vi "gas flow controller -- Pgg3.vi"(5 "gas flow, %":dbl=11.0, 6 "action":T3=enum."stop UP/DOWN", 7 "heater":dbl=11.0, 8 "gas flow controller ref in":refnum<vi>, 10 "seconds":dbl=1.0) -> (0 "gas flow controller out":T1={"UP step (%)"=10.0, "ramp DOWN"=TRUE, "ramp UP"=TRUE, "idle"=TRUE, "UP time (min)"=10.0, "ramp step (%)"=10.0, "check (min)"=10.0, "DOWN step (%)"=10.0, "DOWN time (min)"=10.0, "to"=10.0, "last (min)"=10.0, "below"=TRUE, "above"=TRUE, "Control Gas"=TRUE, "upper"=10.0, "lower"=10.0, "heater"=10.0, "in range"=TRUE, "gas, %"=10.0, "ramp Up progress"={"(total # of ramp steps)"=30, "ramp time step (sec)"=120, "steps so far"=0, "state"=enum."ramp down"}, "ramp Down progress"={"(total # of ramp steps)"=30, "ramp time step (sec)"=120, "steps so far"=0, "state"=enum."ramp down"}, "state"=enum."normal", "set gas"=TRUE})   [LabVIEW 2015]
uses:
  gas flow controller action.ctl
  gas flow controller control -- Pgg2.ctl
  gas flow control - progress.ctl
  gas flow controller state.ctl
  stack action -- control.ctl
  itc 503 box - control.ctl
  Q - not nan -- real.vi
  Q - not nan -- integer.vi
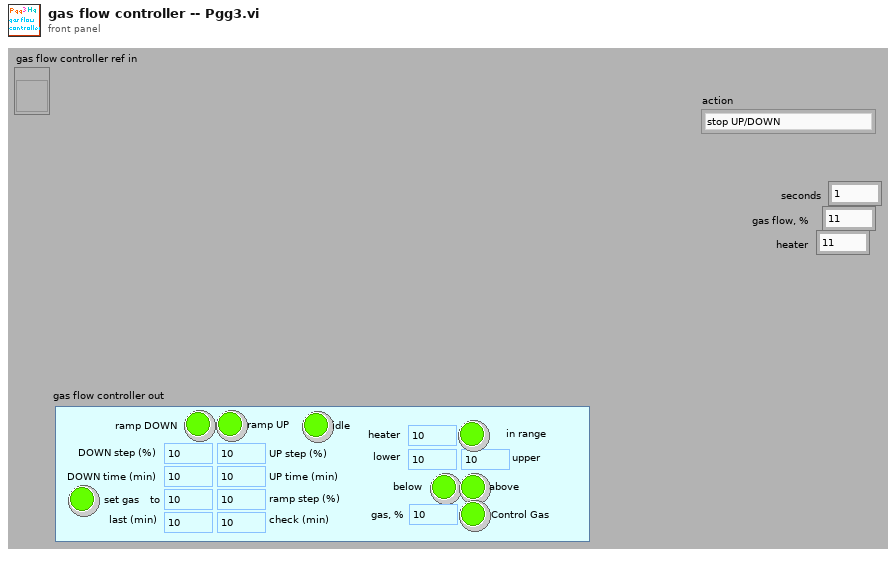
[diagram p1: front panel]
types:
  T1 = typedef "gas flow controller control -- Pgg2.ctl" = cluster{"UP step (%)":dbl, "ramp DOWN":bool, "ramp UP":bool, "idle":bool, "UP time (min)":dbl, "ramp step (%)":dbl, "check (min)":dbl, "DOWN step (%)":dbl, "DOWN time (min)":dbl, "to":dbl, "last (min)":dbl, "below":bool, "above":bool, "Control Gas":bool, "upper":dbl, "lower":dbl, "heater":dbl, "in range":bool, "gas, %":dbl, "ramp Up progress":T2, "ramp Down progress":T2, "state":enum16{"normal", "ramp up", "ramp down"}, "set gas":bool}
  T2 = typedef "gas flow control - progress.ctl" = cluster{"(total # of ramp steps)":i32, "ramp time step (sec)":i32, "steps so far":i32, "state":enum16{"normal", "ramp up", "ramp down"}}
  T3 = typedef "gas flow controller action.ctl" = enum16{"check", "force UP", "stop UP/DOWN", "force DOWN", "init", "set gas to", "turn off", "turn on", "idle", "update parameters", "parse", "set gas"}
  T4 = typedef "gas flow controller state.ctl" = enum16{"normal", "ramp up", "ramp down"}
  T5 = typedef "stack action -- control.ctl" = enum16{"push", "pop", "check", "init"}
  T6 = typedef "itc 503 box - control.ctl" = enum16{"heater manual and zero", "heater auto", "upload D", "upload I", "upload P", "shut off", "init", "read sweep table", "disable", "enable", "read state", "set gas to", "stop sweep", "start sweep", "test", "set temperature to", "write sweep table", "-void", "set heater to"}
  T7 = typedef "comparison control.ctl" = enum16{"not a number", "above", "in range", "below"}
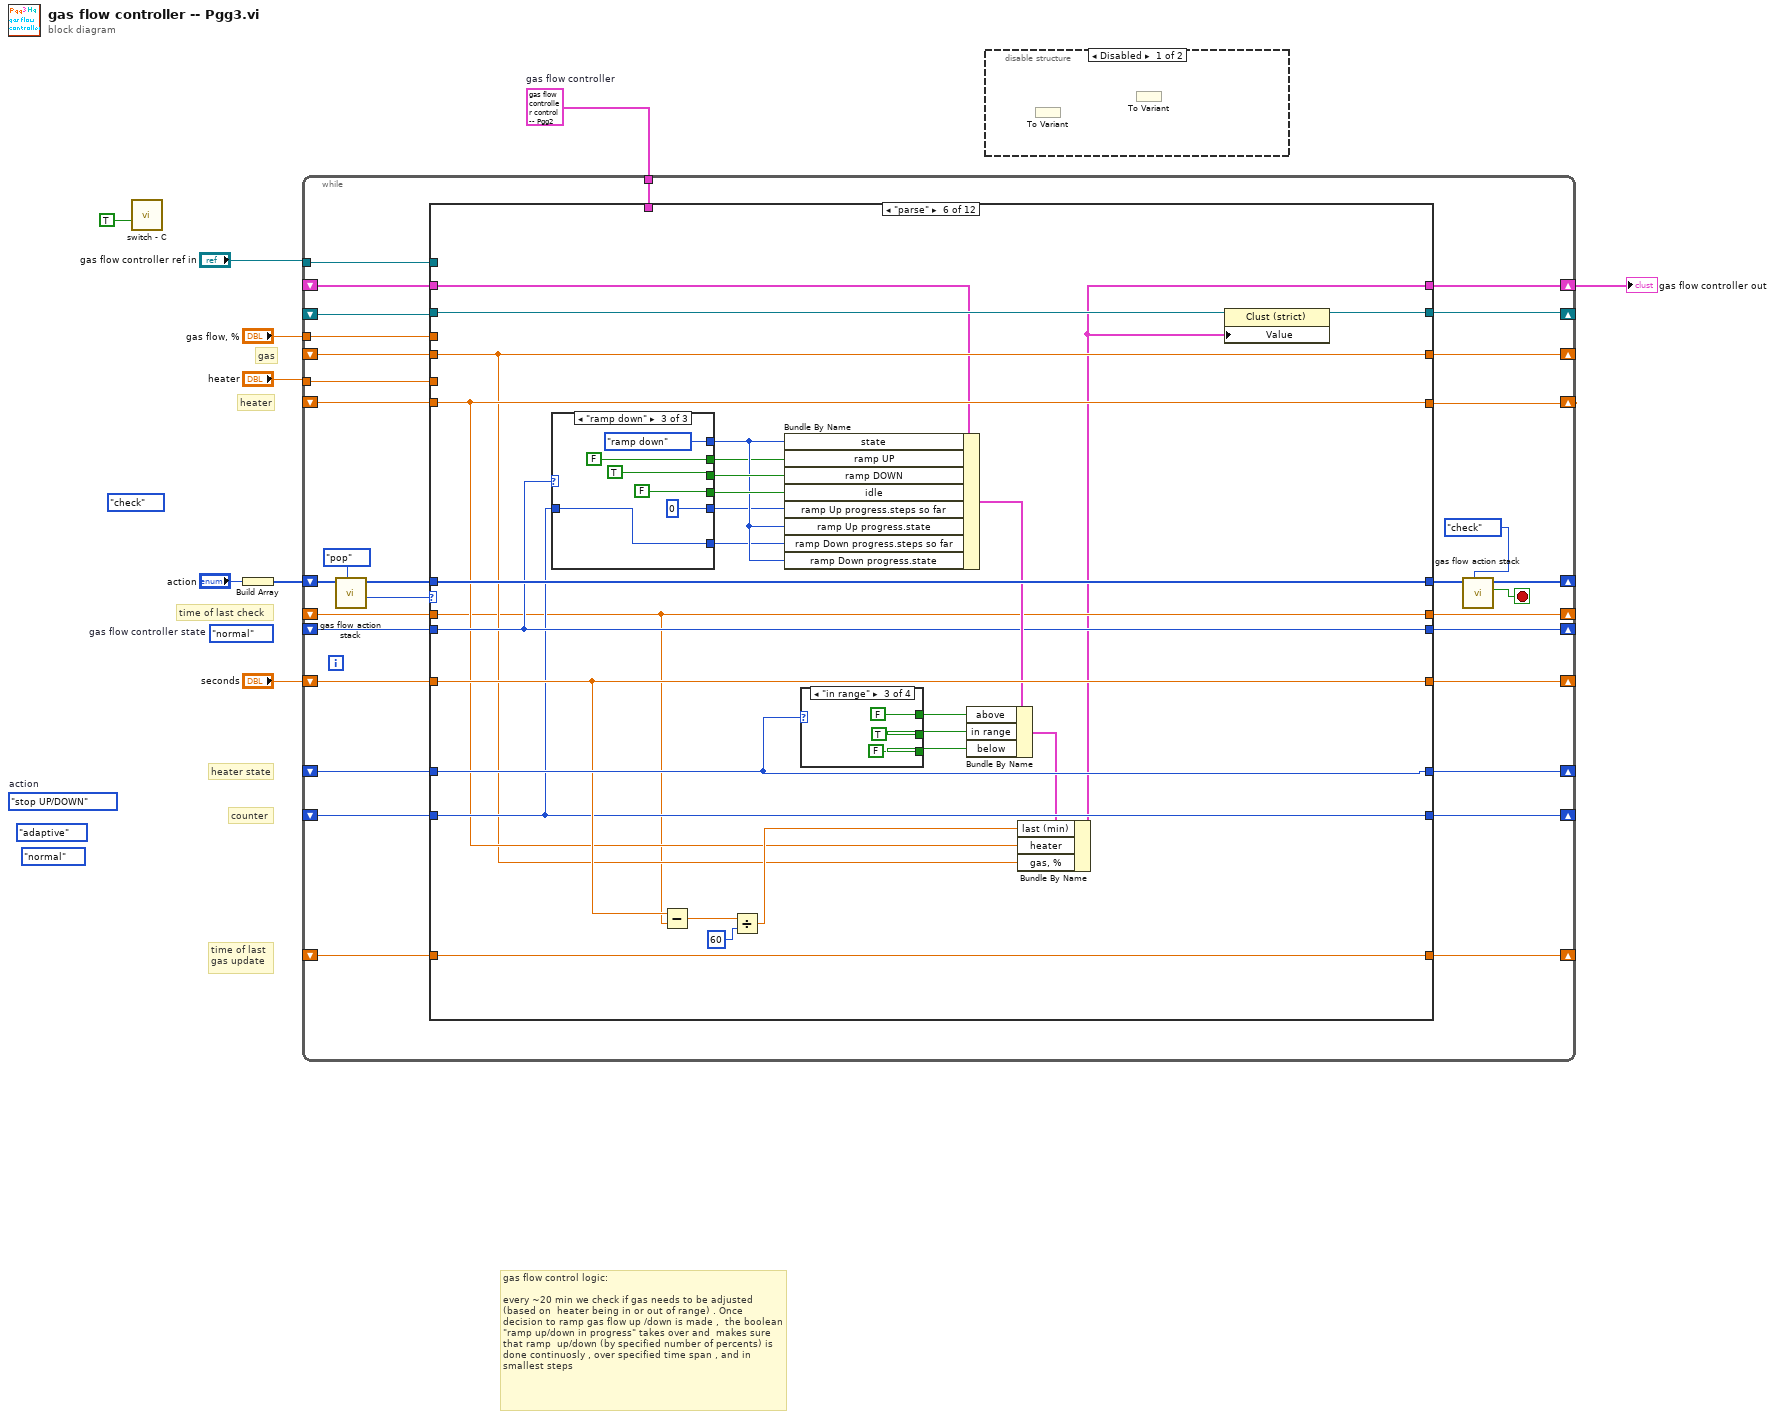
[diagram p0: block diagram]
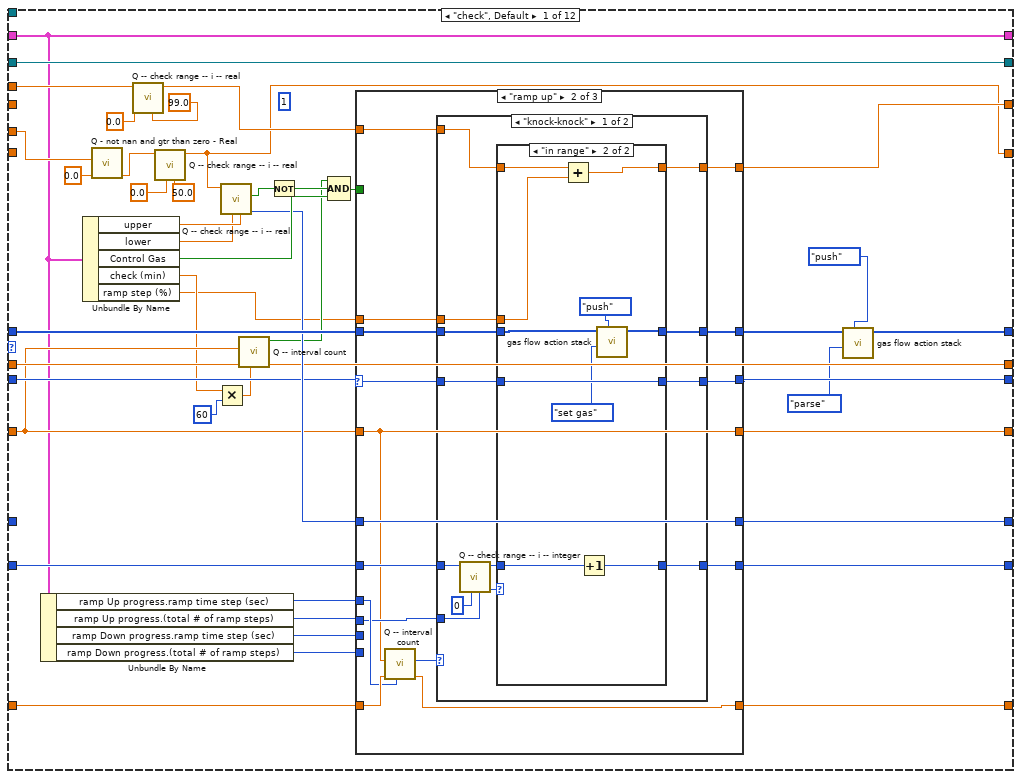
[diagram p3: hidden frame]
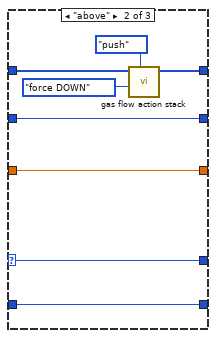
[diagram p6: hidden frame]
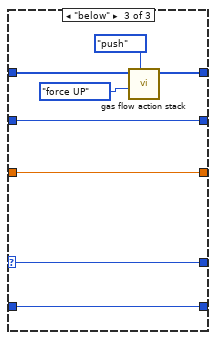
[diagram p7: hidden frame]
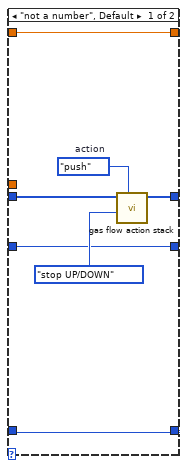
[diagram p8: hidden frame]
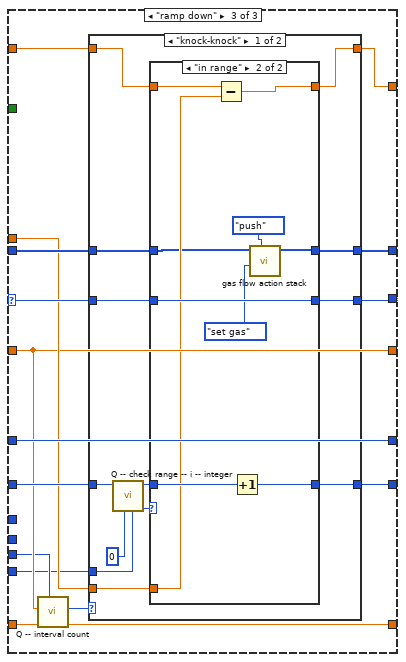
[diagram p10: hidden frame]
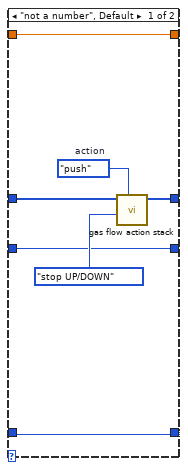
[diagram p11: hidden frame]
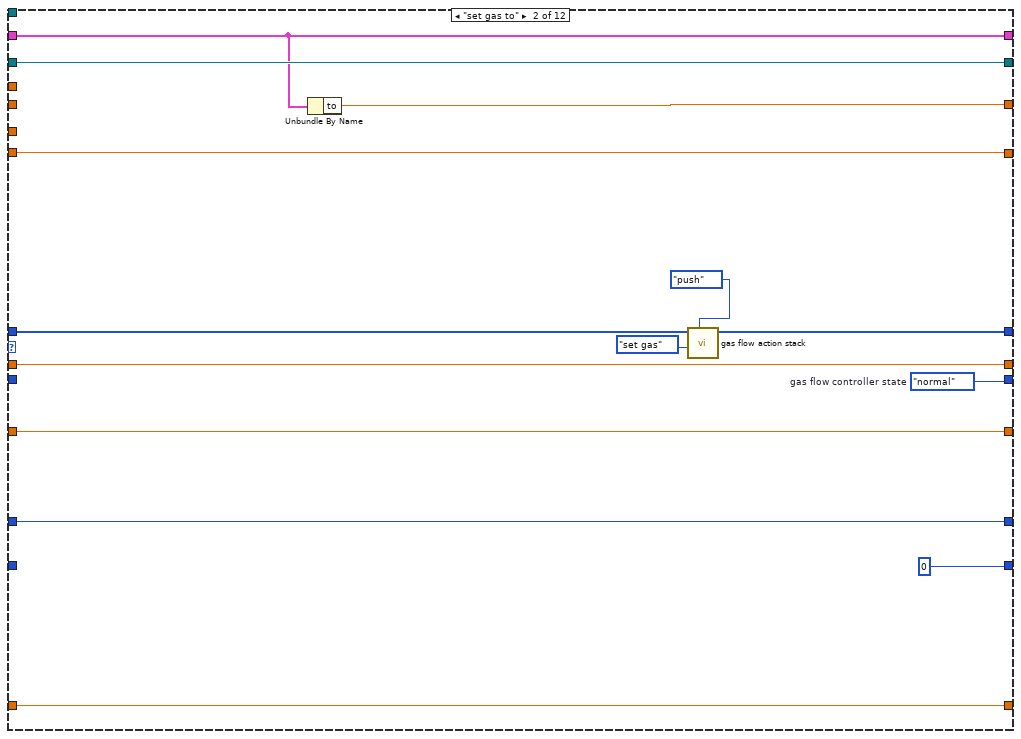
[diagram p13: hidden frame]
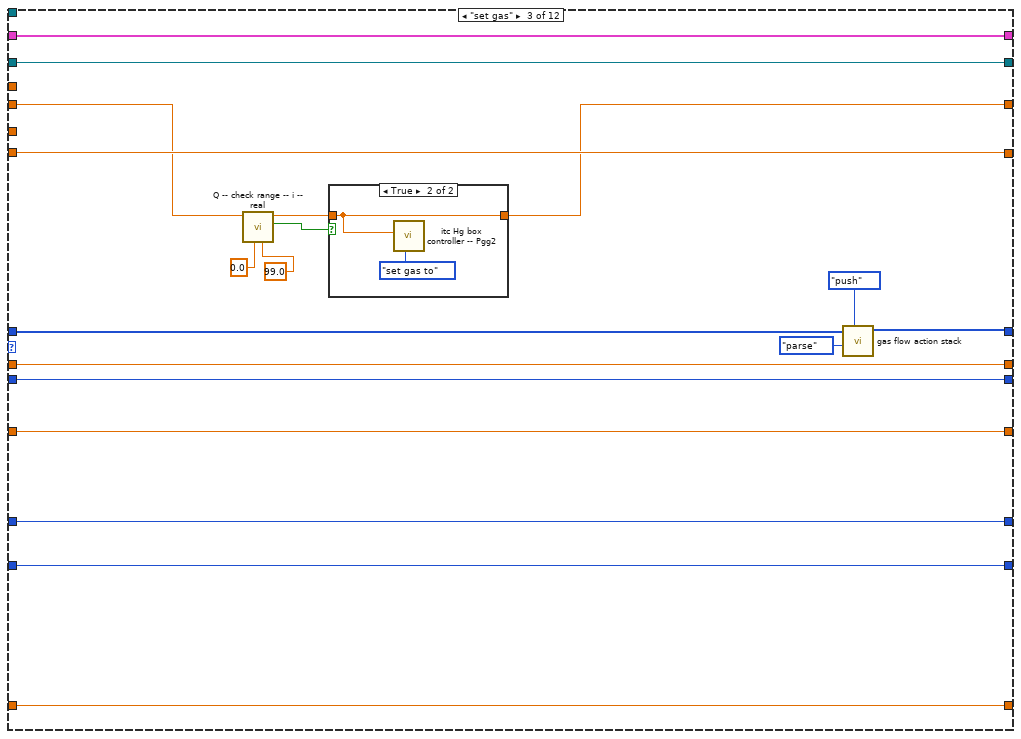
[diagram p14: hidden frame]
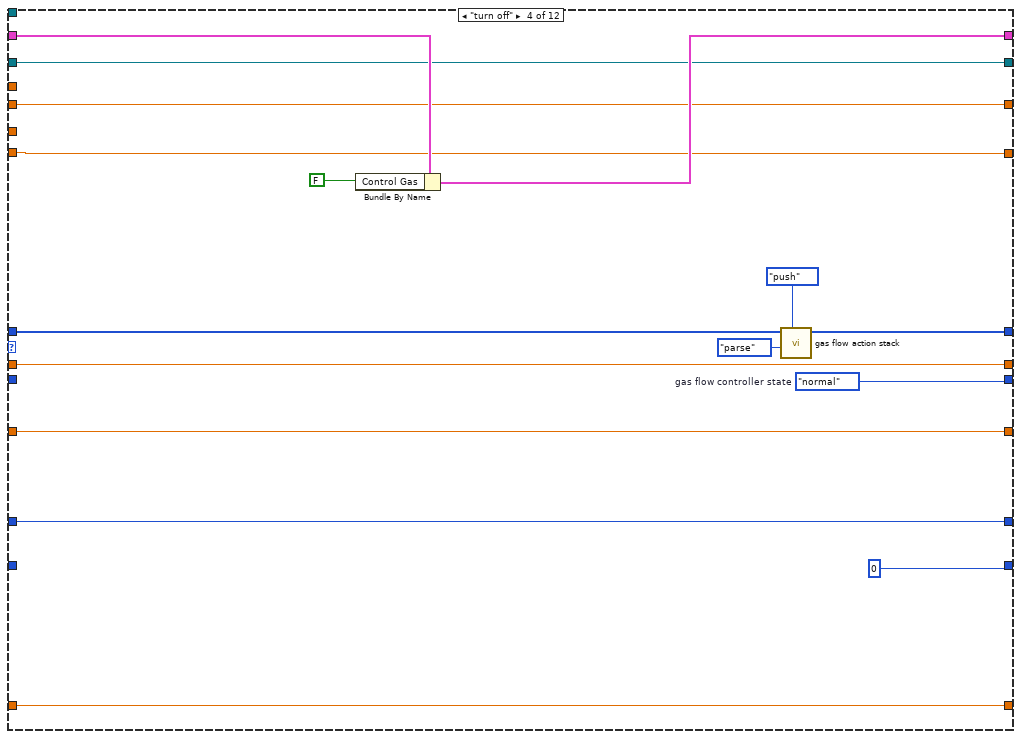
[diagram p16: hidden frame]
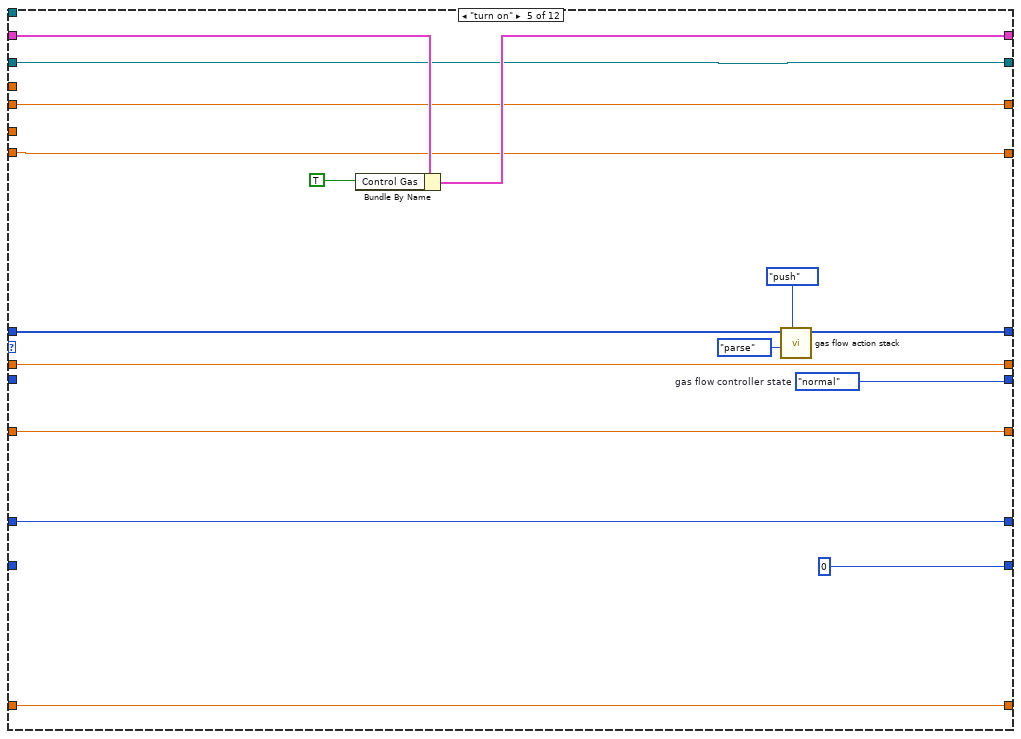
[diagram p17: hidden frame]
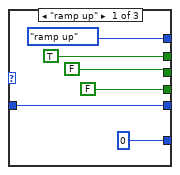
[diagram p18: hidden frame]
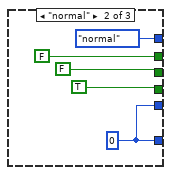
[diagram p19: hidden frame]
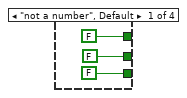
[diagram p20: hidden frame]
diagram:
  (unwired) gas_flow_controller_action."check" ("action")
  w2 = T1 {"UP step (%)"=0.5, "ramp DOWN"=FALSE, "ramp UP"=FALSE, "idle"=FALSE, "UP time (min)"=20.0, "ramp step (%)"=0.1, "check (min)"=3.0, "DOWN step (%)"=0.5, "DOWN time (min)"=20.0, "to"=1.0, "last (min)"=0.0, "below"=FALSE, "above"=FALSE, "Control Gas"=FALSE, "upper"=7.0, "lower"=3.0, "heater"=0.0, "in range"=TRUE, "gas, %"=1.0, "ramp Up progress"={"(total # of ramp steps)"=30, "ramp time step (sec)"=120, "steps so far"=0, "state"=enum."ramp down"}, "ramp Down progress"={"(total # of ramp steps)"=30, "ramp time step (sec)"=120, "steps so far"=0, "state"=enum."ramp down"}, "state"=enum."ramp down", "set gas"=FALSE}  # gas flow controller
  (unwired) enum16{"normal", "ramp up", "ramp down"}."normal" ("state")
  (unwired) enum16{"first time", "uniform", "adaptive"}."adaptive" ("mode")
  (unwired) gas_flow_controller_state."normal"  # gas flow controller state
  (unwired) gas_flow_controller_action."stop UP/DOWN"  # action
  # "heater"
  # "time of last\ngas update"
  # "counter"
  # "heater state"
  # "gas"
  # "gas flow control logic: \n\nevery ~20 min we check if gas needs to be adjusted  (based on  heater being in or out of range) . Once  decision to ramp gas flow up /down is made ,  the boolean \"ramp up/down in progress\" takes over and  makes sure that ramp  up/down (by specified number of percents) is done continuosly , over specified time span , and in smallest steps"
  # "time of last check"
  n1 = call "switch - C.vi"("switch"=TRUE) -> ()  [unwired: 10 in, 1 out]
  n2 = Build Array("action") -> (w5:T3[])
  n3 = while {
    shift-right: [w11] -> w3
    shift-left: _ -> [w41]
    shift-right: [w23] -> _
    shift-left: _ -> [w20]
    tunnel: "gas flow, %" -> [w24]
    tunnel: "heater" -> [w40]
    shift-right: [w38] -> _
    shift-left: _ -> [w37]
    shift-right: [w36] -> _
    shift-left: _ -> [w35]
    shift-right: [w29] -> _
    shift-left: w5 -> [w34]
    shift-right: [w25] -> _
    shift-left: _ -> [w26]
    shift-right: [w22] -> _
    shift-left: _ -> [w21]
    shift-right: [w18] -> _
    shift-left: "seconds" -> [w39]
    shift-right: [w19] -> _
    shift-left: _ -> [w13]
    shift-right: [w17] -> _
    shift-left: _ -> [w16]
    shift-right: [w15] -> _
    shift-left: _ -> [w14]
    tunnel: "gas flow controller ref in" -> [w12]
    tunnel: w2 -> [w10]
    stop <- w27 stop-if-true
    n4 = call "gas flow action stack.vi"("action"=stack_action_--_control."pop", "command stack"=w34) -> ("selector out"=w33:T3, "command stack out"=w31:T3[])  [unwired: 7 in, 1 out]
    n5 = case shown="\"parse\"" w33 {
      tunnel: [w44 w238 w250 w283 w299 w304 w360 w411 w417 w437 w454 w469] -> w11
      tunnel: w41 -> [w44 w238 w250 w286 w302 w305 w369 w411 _ w437 w454 w469]
      tunnel: w40 -> [w49 _ _ _ _ _ _ _ _ _ _ _]
      tunnel: w39 -> [w66 w241 w265 w276 w292 w326 w375 w408 w421 w438 w443 w461]
      tunnel: [w55 w249 w268 w272 w288 w329 w380 w412 w420 w436 w455 w470] -> w38
      tunnel: w37 -> [w55 w249 w268 w272 w288 w308 w368 w412 _ w436 w455 w470]
      tunnel: [w75 w248 w267 w285 w301 w306 w378 w415 w431 w442 w445 w459] -> w36
      tunnel: w35 -> [w77 w248 w267 w285 w301 w306 w378 w415 w431 w442 _ _]
      tunnel: [w59 w245 w260 w281 w297 w330 w377 w403 w424 w435 w448 w463] -> w30
      tunnel: w31 -> [w80 w237 w259 w280 w296 w330 w377 w404 w425 w435 w449 w464]
      tunnel: w26 -> [w78 _ w257 _ _ w317 w376 _ _ w432 _ _]
      tunnel: [w72 w247 w257 w284 w300 w317 w376 w414 w430 w432 w457 w472] -> w25
      tunnel: w24 -> [w71 _ _ _ _ _ _ _ _ _ _ _]
      tunnel: [w51 w246 w251 w278 w294 w309 w370 w410 w428 w441 w453 w468] -> w23
      tunnel: [w50 w242 w266 w277 w293 w310 w371 w409 w427 w440 w452 w467] -> w22
      tunnel: w21 -> [_ w242 w266 w277 w293 w310 w371 w409 w427 w440 w452 w467]
      tunnel: w20 -> [_ _ w253 w278 w294 w309 w370 w410 w428 w441 w453 w468]
      tunnel: [w56 w240 w264 w275 w291 w328 w374 w407 w422 w439 w451 w466] -> w19
      tunnel: [w57 w241 w265 w276 w292 w326 w375 w408 w421 w438 w443 w461] -> w18
      tunnel: [w65 w239 w262 w274 w290 w327 w372 w405 w421 w434 w445 w459] -> w17
      tunnel: w16 -> [w64 w239 w262 w274 w290 w327 w372 w405 _ w434 w444 w458]
      tunnel: [w63 0 w263 0 0 w314 w373 0 0 w433 0 0] -> w15
      tunnel: w14 -> [w62 _ w263 _ _ w314 w373 _ _ w433 _ _]
      tunnel: w13 -> [_ w240 w264 w275 w291 w328 w374 w407 w422 w439 w451 w466]
      tunnel: w12 -> [_ _ _ _ _ _ _ _ w419 _ _ _]
      tunnel: w10 -> [_ _ _ _ _ _ w361 _ w416 _ _ _]
      frame "check", Default {
        (unwired) 1
        n6 = Unbundle By Name(w44) -> ("ramp Up progress.ramp time step (sec)"=w54:i32, "ramp Up progress.(total # of ramp steps)"=w53:i32, "ramp Down progress.ramp time step (sec)"=w46:i32, "ramp Down progress.(total # of ramp steps)"=w45:i32)
        n7 = Unbundle By Name(w44) -> ("upper"=w84:dbl, "lower"=w83:dbl, "Control Gas"=w86:bool, "check (min)"=w43:dbl, "ramp step (%)"=w42:dbl)
        n8 = call "Q - not nan and gtr than zero - Real.vi"("default"=0.0 ("y"), "Numeric"=w49) -> ("out"=w47:dbl)  [unwired: 8 in, 1 out]
        n9 = call "Q -- check range -- i -- real.vi"("upper"=99.0 ("y"), "lower"=0.0 ("y"), "number"=w71) -> ("number in range"=w52:dbl)  [unwired: 6 in, 2 out]
        n10 = call "Q -- check range -- i -- real.vi"("upper"=50.0 ("y"), "lower"=0.0 ("y"), "number"=w47) -> ("number in range"=w50:dbl)  [unwired: 6 in, 2 out]
        n11 = Multiply(x=w43, y=60) -> (x*y=w76:dbl)
        n12 = call "Q -- check range -- i -- real.vi"("upper"=w84, "lower"=w83, "number"=w50) -> ("selector"=w79:T7, "in range?"=w82:bool)  [unwired: 6 in, 1 out]
        n13 = call "Q -- interval count.vi"("interval (sec)"=w76, "last time (sec)"=w77, "current time (sec)"=w66) -> ("last time out (sec)"=w75:dbl, "tic"=w73:bool)  [unwired: 5 in, 2 out]
        n14 = Not(x=w82) -> (.not. x?=w85:bool)
        n15 = Compound Arithmetic op=AND(w73, w85, w86) -> (w81:bool)
        n16 = case shown="\"ramp up\"" w78 {
          selector: w78 -> [w92 w144 w194]
          tunnel: w81 -> [w99 _ _]
          tunnel: w66 -> [w98 w136 w188]
          tunnel: [w87 w150 w200] -> w65
          tunnel: w64 -> [w87 w151 w201]
          tunnel: [w97 w147 w197] -> w60
          tunnel: w80 -> [w96 w146 w196]
          tunnel: w79 -> [w95 w142 w192]
          tunnel: [w94 w145 w195] -> w72
          tunnel: [w93 w148 w198] -> w63
          tunnel: w62 -> [w89 w149 w199]
          tunnel: [w91 w136 w188] -> w57
          tunnel: [w90 w142 w192] -> w56
          tunnel: w54 -> [_ w141 _]
          tunnel: w53 -> [_ w140 _]
          tunnel: w52 -> [w88 w139 w191]
          tunnel: w42 -> [_ w138 w190]
          tunnel: [w88 w137 w189] -> w51
          tunnel: w46 -> [_ _ w187]
          tunnel: w45 -> [_ _ w186]
          frame "normal", Default {
            n17 = case shown="False" w99 {
              tunnel: w98 -> [w102 w109]
              tunnel: [w104 w112] -> w97
              tunnel: w96 -> [w104 w113]
              tunnel: w95 -> [w101 w114]
              tunnel: [w103 w111] -> w94
              tunnel: w92 -> [w103 w110]
              tunnel: [w100 w108] -> w93
              tunnel: [w102 w107] -> w91
              tunnel: [w101 w106] -> w90
              tunnel: w89 -> [w100 w105]
              frame False {
              }
              frame True {
                n18 = case shown="\"not a number\", Default" w114 {
                  selector: w114 -> [w115 w121 w129]
                  tunnel: w113 -> [w119 w126 w134]
                  tunnel: [w119 w125 w133] -> w112
                  tunnel: [w118 w123 w131] -> w111
                  tunnel: w110 -> [w118 w123 w131]
                  tunnel: [w117 w122 w130] -> w107
                  tunnel: w109 -> [w117 w122 w130]
                  tunnel: [w116 w120 w128] -> w108
                  tunnel: [w115 w121 w129] -> w106
                  tunnel: w105 -> [w116 w120 w128]
                  frame "not a number", Default {
                  }
                  frame "above" {
                    n19 = call "gas flow action stack.vi"("action"=stack_action_--_control."push", "selector in"=gas_flow_controller_action."force DOWN" ("selector"), "command stack"=w126) -> ("command stack out"=w125:T3[])  [unwired: 6 in, 2 out]
                  }
                  frame "below" {
                    n20 = call "gas flow action stack.vi"("action"=stack_action_--_control."push", "selector in"=gas_flow_controller_action."force UP" ("selector"), "command stack"=w134) -> ("command stack out"=w133:T3[])  [unwired: 6 in, 2 out]
                  }
                }
              }
            }
          }
          frame "ramp up" {
            n21 = call "Q -- interval count.vi"("interval (sec)"=w141, "last time (sec)"=w151, "current time (sec)"=w136) -> ("last time out (sec)"=w150:dbl, "tic state"=w143:enum16{"knock-knock", "none"})  [unwired: 5 in, 2 out]
            n22 = case shown="\"knock-knock\"" w143 {
              tunnel: w149 -> [w156 w183]
              tunnel: [w160 w183] -> w148
              tunnel: [w164 w185] -> w147
              tunnel: w146 -> [w163 w185]
              tunnel: [w162 w184] -> w145
              tunnel: w144 -> [w161 w184]
              tunnel: w140 -> [w155 _]
              tunnel: w139 -> [w154 w182]
              tunnel: w138 -> [w153 _]
              tunnel: [w152 w182] -> w137
              frame "knock-knock" {
                n23 = call "Q -- check range -- i -- integer.vi"("upper"=w155, "lower"=0, "number"=w156) -> ("selector"=w158:T7, "number in range"=w157:i32)  [unwired: 6 in, 1 out]
                n24 = case shown="\"in range\"" w158 {
                  tunnel: [w169 w173] -> w164
                  tunnel: w163 -> [w170 w174]
                  tunnel: [w167 w181] -> w162
                  tunnel: w161 -> [w167 w181]
                  tunnel: w157 -> [w166 w180]
                  tunnel: [w166 w179] -> w160
                  tunnel: w154 -> [w165 w178]
                  tunnel: w153 -> [_ w177]
                  tunnel: [w165 w176] -> w152
                  frame "not a number", Default {
                    w171 = stack_action_--_control."push"  # action
                    n25 = call "gas flow action stack.vi"("action"=w171, "selector in"=gas_flow_controller_action."stop UP/DOWN" ("selector"), "command stack"=w170) -> ("command stack out"=w169:T3[])  [unwired: 6 in, 2 out]
                  }
                  frame "in range" {
                    n26 = Add(x=w178, y=w177) -> (x+y=w176:dbl)
                    n27 = Increment(x=w180) -> (x+1=w179:i32)
                    n28 = call "gas flow action stack.vi"("action"=stack_action_--_control."push", "selector in"=gas_flow_controller_action."set gas" ("selector"), "command stack"=w174) -> ("command stack out"=w173:T3[])  [unwired: 6 in, 2 out]
                  }
                }
              }
              frame "none", Default {
              }
            }
          }
          frame "ramp down" {
            n29 = call "Q -- interval count.vi"("interval (sec)"=w187, "last time (sec)"=w201, "current time (sec)"=w188) -> ("last time out (sec)"=w200:dbl, "tic state"=w193:enum16{"knock-knock", "none"})  [unwired: 5 in, 2 out]
            n30 = case shown="\"knock-knock\"" w193 {
              tunnel: w199 -> [w206 w233]
              tunnel: [w210 w233] -> w198
              tunnel: [w214 w235] -> w197
              tunnel: w196 -> [w213 w235]
              tunnel: [w212 w234] -> w195
              tunnel: w194 -> [w211 w234]
              tunnel: w186 -> [w205 _]
              tunnel: w191 -> [w204 w232]
              tunnel: w190 -> [w203 _]
              tunnel: [w202 w232] -> w189
              frame "knock-knock" {
                n31 = call "Q -- check range -- i -- integer.vi"("upper"=w205, "lower"=0, "number"=w206) -> ("selector"=w208:T7, "number in range"=w207:i32)  [unwired: 6 in, 1 out]
                n32 = case shown="\"in range\"" w208 {
                  tunnel: [w219 w223] -> w214
                  tunnel: w213 -> [w220 w224]
                  tunnel: [w217 w231] -> w212
                  tunnel: w211 -> [w217 w231]
                  tunnel: w207 -> [w216 w230]
                  tunnel: [w216 w229] -> w210
                  tunnel: w204 -> [w215 w228]
                  tunnel: w203 -> [_ w227]
                  tunnel: [w215 w226] -> w202
                  frame "not a number", Default {
                    w221 = stack_action_--_control."push"  # action
                    n33 = call "gas flow action stack.vi"("action"=w221, "selector in"=gas_flow_controller_action."stop UP/DOWN" ("selector"), "command stack"=w220) -> ("command stack out"=w219:T3[])  [unwired: 6 in, 2 out]
                  }
                  frame "in range" {
                    n34 = Subtract(x=w228, y=w227) -> (x-y=w226:dbl)
                    n35 = Increment(x=w230) -> (x+1=w229:i32)
                    n36 = call "gas flow action stack.vi"("action"=stack_action_--_control."push", "selector in"=gas_flow_controller_action."set gas" ("selector"), "command stack"=w224) -> ("command stack out"=w223:T3[])  [unwired: 6 in, 2 out]
                  }
                }
              }
              frame "none", Default {
              }
            }
          }
        }
        n37 = call "gas flow action stack.vi"("action"=stack_action_--_control."push", "selector in"=gas_flow_controller_action."parse" ("selector"), "command stack"=w60) -> ("command stack out"=w59:T3[])  [unwired: 6 in, 2 out]
      }
      frame "set gas to" {
        w247 = gas_flow_controller_state."normal"  # gas flow controller state
        n38 = Unbundle By Name(w238) -> ("to"=w246:dbl)
        n39 = call "gas flow action stack.vi"("action"=stack_action_--_control."push", "selector in"=gas_flow_controller_action."set gas" ("selector"), "command stack"=w237) -> ("command stack out"=w245:T3[])  [unwired: 6 in, 2 out]
      }
      frame "set gas" {
        n40 = call "Q -- check range -- i -- real.vi"("upper"=99.0 ("y"), "lower"=0.0 ("y"), "number"=w253) -> ("in range?"=w254:bool, "number in range"=w252:dbl)  [unwired: 6 in, 1 out]
        n41 = case shown="True" w254 {
          tunnel: [w269 w270] -> w251
          tunnel: w252 -> [w269 w270]
          frame False {
          }
          frame True {
            n42 = call "itc Hg box controller -- Pgg2.vi"("itc box action"=itc_503_box_-_control."set gas to", "input"=w270) -> ()  [unwired: 7 in, 3 out]
          }
        }
        n43 = call "gas flow action stack.vi"("action"=stack_action_--_control."push", "selector in"=gas_flow_controller_action."parse" ("selector"), "command stack"=w259) -> ("command stack out"=w260:T3[])  [unwired: 6 in, 2 out]
      }
      frame "turn off" {
        w284 = gas_flow_controller_state."normal"  # gas flow controller state
        n44 = Bundle By Name(cluster=w286, "Control Gas"=FALSE) -> (w283:T1)
        n45 = call "gas flow action stack.vi"("action"=stack_action_--_control."push", "selector in"=gas_flow_controller_action."parse" ("selector"), "command stack"=w280) -> ("command stack out"=w281:T3[])  [unwired: 6 in, 2 out]
      }
      frame "turn on" {
        w300 = gas_flow_controller_state."normal"  # gas flow controller state
        n46 = Bundle By Name(cluster=w302, "Control Gas"=TRUE) -> (w299:T1)
        n47 = call "gas flow action stack.vi"("action"=stack_action_--_control."push", "selector in"=gas_flow_controller_action."parse" ("selector"), "command stack"=w296) -> ("command stack out"=w297:T3[])  [unwired: 6 in, 2 out]
      }
      frame "parse" {
        n48 = case shown="\"ramp down\"" w317 {
          tunnel: [TRUE FALSE FALSE] -> w307
          tunnel: [FALSE FALSE TRUE] -> w323
          tunnel: [FALSE TRUE FALSE] -> w322
          tunnel: [enum16{"normal", "ramp up", "ramp down"}."ramp up" ("state") enum16{"normal", "ramp up", "ramp down"}."normal" ("state") enum16{"normal", "ramp up", "ramp down"}."ramp down" ("state")] -> w316
          tunnel: [0 w337 w342] -> w313
          tunnel: [w332 w337 0] -> w315
          tunnel: w314 -> [w332 _ w342]
          frame "ramp up" {
          }
          frame "normal" {
            w337 = 0
          }
          frame "ramp down" {
          }
        }
        n49 = Subtract(x=w326, y=w306) -> (x-y=w324:dbl)
        n50 = Divide(x=w324, y=60) -> (x/y=w311:dbl)
        n51 = Bundle By Name(cluster=w305, "state"=w316, "ramp UP"=w307, "ramp DOWN"=w323, "idle"=w322, "ramp Up progress.steps so far"=w315, "ramp Up progress.state"=w316, "ramp Down progress.steps so far"=w313, "ramp Down progress.state"=w316) -> (w318:T1)
        n52 = case shown="\"in range\"" w328 {
          tunnel: [FALSE TRUE FALSE FALSE] -> w321
          tunnel: [FALSE FALSE TRUE FALSE] -> w320
          tunnel: [FALSE FALSE FALSE TRUE] -> w319
          frame "not a number", Default {
          }
          frame "above" {
          }
          frame "in range" {
          }
          frame "below" {
          }
        }
        n53 = Bundle By Name(cluster=w318, "above"=w321, "in range"=w320, "below"=w319) -> (w312:T1)
        n54 = Bundle By Name(cluster=w312, "last (min)"=w311, "heater"=w310, "gas, %"=w309) -> (w304:T1)
        n55 = property class="Clust (strict)"(reference=w308, "Value"=w304) -> (reference out=w329:refnum<vi>)  [unwired: 1 in, 1 out]
      }
      frame "update parameters" {
        # "update  parameters"
        n56 = property class="Clust (strict)"(reference=w368) -> (reference out=w367:refnum<vi>, "Value"=w366:T1)  [unwired: 1 in, 1 out]
        n57 = Variant To Data(type=w361, Variant=w366) -> (data=w364:T1)  [unwired: 1 in, 1 out]
        n58 = Unbundle By Name(w364) -> ("DOWN step (%)"=w387:dbl, "DOWN time (min)"=w386:dbl)
        n59 = Unbundle By Name(w364) -> ("ramp step (%)"=w363:dbl)
        n60 = Unbundle By Name(w364) -> ("UP step (%)"=w379:dbl, "UP time (min)"=w388:dbl)
        n61 = Divide(x=w379, y=w363) -> (x/y=w401:dbl)
        n62 = Divide(x=w387, y=w363) -> (x/y=w394:dbl)
        n63 = Multiply(x=w388, y=60) -> (x*y=w399:dbl)
        n64 = Multiply(x=w386, y=60) -> (x*y=w392:dbl)
        n65 = Round Toward +Infinity(x=w399) -> (ceil(x): smallest int >= x=w398:dbl)
        n66 = Round Toward +Infinity(x=w401) -> (ceil(x): smallest int >= x=w400:dbl)
        n67 = Round Toward +Infinity(x=w394) -> (ceil(x): smallest int >= x=w393:dbl)
        n68 = Round Toward +Infinity(x=w392) -> (ceil(x): smallest int >= x=w391:dbl)
        n69 = To Long Integer(number=w398) -> (32bit integer=w396:i32)
        n70 = To Long Integer(number=w400) -> (32bit integer=w395:i32)
        n71 = To Long Integer(number=w393) -> (32bit integer=w384:i32)
        n72 = To Long Integer(number=w391) -> (32bit integer=w389:i32)
        n73 = Unbundle By Name(w364) -> ("to"=w383:dbl, "upper"=w382:dbl, "lower"=w381:dbl, "check (min)"=w362:dbl)
        n74 = Quotient & Remainder(x=w396, y=w395) -> (floor(x/y)=w365:i32)  [unwired: 1 out]
        n75 = Quotient & Remainder(x=w389, y=w384) -> (floor(x/y)=w385:i32)  [unwired: 1 out]
        n76 = Bundle By Name(cluster=w369, "ramp Up progress.(total # of ramp steps)"=w395, "ramp Up progress.ramp time step (sec)"=w365, "UP step (%)"=w379, "UP time (min)"=w388, "ramp step (%)"=w363, "DOWN step (%)"=w387, "DOWN time (min)"=w386, "ramp Down progress.(total # of ramp steps)"=w384, "ramp Down progress.ramp time step (sec)"=w385, "to"=w383, "upper"=w382, "lower"=w381, "check (min)"=w362) -> (w360:T1)
        n77 = property class="Clust (strict)"(reference=w367, "Value"=w360) -> (reference out=w380:refnum<vi>)  [unwired: 1 in, 1 out]
      }
      frame "stop UP/DOWN" {
        w414 = gas_flow_controller_state."normal"  # gas flow controller state
        n78 = call "gas flow action stack.vi"("action"=stack_action_--_control."push", "selector in"=gas_flow_controller_action."parse" ("selector"), "command stack"=w404) -> ("command stack out"=w403:T3[])  [unwired: 6 in, 2 out]
      }
      frame "init" {
        w430 = gas_flow_controller_state."normal"  # gas flow controller state
        n79 = property class="Clust (strict)"(reference=w419) -> (reference out=w420:refnum<vi>, "Value"=w418:T1)  [unwired: 1 in, 1 out]
        n80 = Variant To Data(type=w416, Variant=w418) -> (data=w417:T1)  [unwired: 1 in, 1 out]
        n81 = call "gas flow action stack.vi"("action"=stack_action_--_control."push", "selector in"=gas_flow_controller_action."parse" ("selector"), "command stack"=w425) -> ("command stack out"=w424:T3[])  [unwired: 6 in, 2 out]
      }
      frame "idle" {
      }
      frame "force DOWN" {
        w457 = gas_flow_controller_state."ramp down"  # gas flow controller state
        n82 = Subtract(x=w444, y=10000) -> (x-y=w445:dbl)
        n83 = call "gas flow action stack.vi"("action"=stack_action_--_control."push", "selector in"=gas_flow_controller_action."parse" ("selector"), "command stack"=w449) -> ("command stack out"=w448:T3[])  [unwired: 6 in, 2 out]
      }
      frame "force UP" {
        w472 = gas_flow_controller_state."ramp up"  # gas flow controller state
        n84 = Subtract(x=w458, y=10000) -> (x-y=w459:dbl)
        n85 = call "gas flow action stack.vi"("action"=stack_action_--_control."push", "selector in"=gas_flow_controller_action."parse" ("selector"), "command stack"=w464) -> ("command stack out"=w463:T3[])  [unwired: 6 in, 2 out]
      }
    }
    n86 = call "gas flow action stack.vi"("action"=stack_action_--_control."check", "command stack"=w30) -> ("stack is empty ?"=w27:bool, "command stack out"=w29:T3[])  [unwired: 7 in, 1 out]
  }
  "gas flow controller out" <- w3
  n87 = disable-structure shown="Disabled" {
    frame Disabled {
      n88 = To Variant() -> ()  [unwired: 1 in, 1 out]
      n89 = To Variant() -> ()  [unwired: 1 in, 1 out]
    }
    frame Enabled {
    }
  }
